vi "ping.vi"(7 "stop":bool, 8 "error in (no error)":errorcluster, 9 "Temperature (deg C)":dbl=25.0, 10 "myRIO DIO Channel":tag="C/DIO1", 11 "Digital in":refnum<vi>) -> (0 "error out":errorcluster, 3 "Distance (cm)":dbl)   [LabVIEW 2017]
uses:
  <vilib>/myRIO/Instrument Drivers/Onboard IO/DIO/typedefs/DIO Reference.ctl
  <vilib>/myRIO/Common/Instrument Driver Framework/Utilities/typedefs/myRIO Generic Hardware Reference.ctl
  <vilib>/myRIO/Common/Instrument Driver Framework/Utilities/typedefs/Hardware Version Enum.ctl
  <vilib>/myRIO/Common/Instrument Driver Framework/Utilities/typedefs/myRIO v1.0 Reference.ctl
  <vilib>/myRIO/Common/Instrument Driver Framework/Utilities/typedefs/Generic FPGA Reference.ctl
  <vilib>/myRIO/Common/Instrument Driver Framework/myRIO v1.0/DIO/typedefs/DIO Channels List.ctl
  <vilib>/myRIO/Common/Instrument Driver Framework/myRIO v1.0/DIO/typedefs/DIO Channels Enum.ctl
  <vilib>/userdefined/High Color/nirio_resource_hc.ctl
  <vilib>/myRIO/Common/Instrument Driver Framework/Utilities/vis/Is FPGA Ref Available.vi
  <vilib>/myRIO/Common/Instrument Driver Framework/myRIO v1.0/DIO/vis/myRIO v1.1 Open DIO.vi
  <vilib>/myRIO/Common/Instrument Driver Framework/Utilities/vis/Validate Channels.vi
  <vilib>/myRIO/Common/Instrument Driver Framework/myRIO v1.0/DIO/vis/myRIO v1.0 Reserve DIO.vi
  <vilib>/myRIO/Common/Instrument Driver Framework/myRIO v1.0/DIO/vis/myRIO v1.0 Close DIO.vi
  <vilib>/myRIO/Common/Instrument Driver Framework/myRIO v1.0/Resource Manager/vis/myRIO v1.0 Reserve Channel List.vi
  <vilib>/myRIO/Common/Instrument Driver Framework/myRIO v1.0/DIO/vis/myRIO v1.0 Build MUX Configuration DIO.vi
  <vilib>/myRIO/Common/Instrument Driver Framework/myRIO v1.0/DIO/vis/myRIO v1.0 Unreserve DIO.vi
  <vilib>/myRIO/Common/Instrument Driver Framework/myRIO v1.0/Resource Manager/vis/myRIO v1.0 Reserve Channel.vi
  <vilib>/myRIO/Common/Instrument Driver Framework/myRIO v1.0/Resource Manager/vis/myRIO v1.0 Unreserve Channel.vi
  <vilib>/myRIO/Common/Instrument Driver Framework/myRIO v1.0/Resource Manager/vis/myRIO v1.0 Create Configuration List.vi
  <vilib>/myRIO/Common/Instrument Driver Framework/myRIO v1.0/Resource Manager/vis/myRIO v1.0 Unreserve Channel List.vi
  <vilib>/myRIO/Common/Instrument Driver Framework/myRIO v1.0/Resource Manager/vis/myRIO v1.0 Build Mutex Name.vi
  <vilib>/Utility/VariantDataType/GetNumericInfo.vi
  <vilib>/Utility/error.llb/Error Cluster From Error Code.vi
  <vilib>/myRIO/Common/Instrument Driver Framework/myRIO v1.0/myRIO v1.1 Open.vi
  <vilib>/myRIO/Common/Instrument Driver Framework/Utilities/vis/IO Manager.vi
  <vilib>/myRIO/Common/Instrument Driver Framework/Utilities/vis/Configuration Manager.vi
  <vilib>/myRIO/Common/Instrument Driver Framework/myRIO v1.0/Resource Manager/vis/myRIO v1.0 Configure IO.vi
  <vilib>/myRIO/Common/Instrument Driver Framework/myRIO v1.0/myRIO v1.0 Close.vi
  <vilib>/myRIO/Common/Instrument Driver Framework/myRIO v1.0/DIO/vis/myRIO v1.0 Write DIO.vi
  <vilib>/myRIO/Common/Instrument Driver Framework/myRIO v1.0/DIO/vis/myRIO v1.0 Read DIO.vi
  <vilib>/myRIO/Common/Instrument Driver Framework/myRIO v1.0/DIO/vis/myRIO v1.0 Shutdown DIO.vi
  <vilib>/myRIO/Express VI/Onboard Devices/LED/LED Express VI.xnode
  <vilib>/myRIO/Instrument Drivers/Onboard IO/DIO/vis/myRIO DIO Open.xnode
  <vilib>/myRIO/Instrument Drivers/Onboard IO/DIO/DIO.lvlib
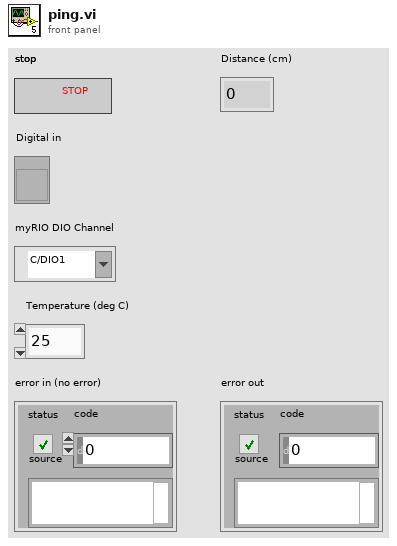
[diagram p1: front panel]
types:
  T1 = enum16{"Initialize", "Trigger pulse", "Wait for rising edge", "Wait for falling edge", "Calculate distance", "Stop"}
  T2 = typedef "DIO.lvlib/DIO Reference.ctl" = cluster{"myRIO Reference":T3, "DIO Channels List":T7}
  T3 = typedef "myRIO Generic Hardware Reference.ctl" = cluster{"myRIO Model":T4, "myRIO Hardware Reference":T5}
  T4 = typedef "Hardware Version Enum.ctl" = enum16{"Unknown", "myRIO-1900", "myRIO-1950", "roboRIO", "NI ELVIS RIO CM"}
  T5 = typedef "myRIO v1.0 Reference.ctl" = cluster{"Generic FPGA Reference":T6, "Allow multiple opens":bool}
  T6 = typedef "Generic FPGA Reference.ctl" = refnum<k20>
  T7 = typedef "DIO Channels List.ctl" = T8[]
  T8 = typedef "DIO Channels Enum.ctl" = enum16{"Not Connected", "C/DIO0", "C/DIO1", "C/DIO2", "C/DIO3", "C/DIO4", "C/DIO5", "C/DIO6", "C/DIO7", "A/DIO0", "A/DIO1", "A/DIO2", "A/DIO3", "A/DIO4", "A/DIO5", "A/DIO6", "A/DIO7", "A/DIO8", "A/DIO9", "A/DIO10", "A/DIO11", "A/DIO12", "A/DIO13", "A/DIO14", "A/DIO15", "B/DIO0", "B/DIO1", "B/DIO2", "B/DIO3", "B/DIO4", "B/DIO5", "B/DIO6", "B/DIO7", "B/DIO8", "B/DIO9", "B/DIO10", "B/DIO11", "B/DIO12", "B/DIO13", "B/DIO14", "B/DIO15", "LED0", "LED1", "LED2", "LED3", "Button0", "DIO/DIO0", "DIO/DIO1", "DIO/DIO2", "DIO/DIO3", "DIO/DIO4", "DIO/DIO5", "DIO/DIO6", "DIO/DIO7", "DIO/DIO8", "DIO/DIO9", "SPI/CS0", "SPI/CS1", "SPI/CS2", "SPI/CS3", "LED RADIO (Green)", "LED RADIO (Red)", "LED COMM (Green)", "LED COMM (Red)", "LED MODE (Green)", "LED MODE (Red)"}
  T9 = typedef "nirio_resource_hc.ctl" = tag
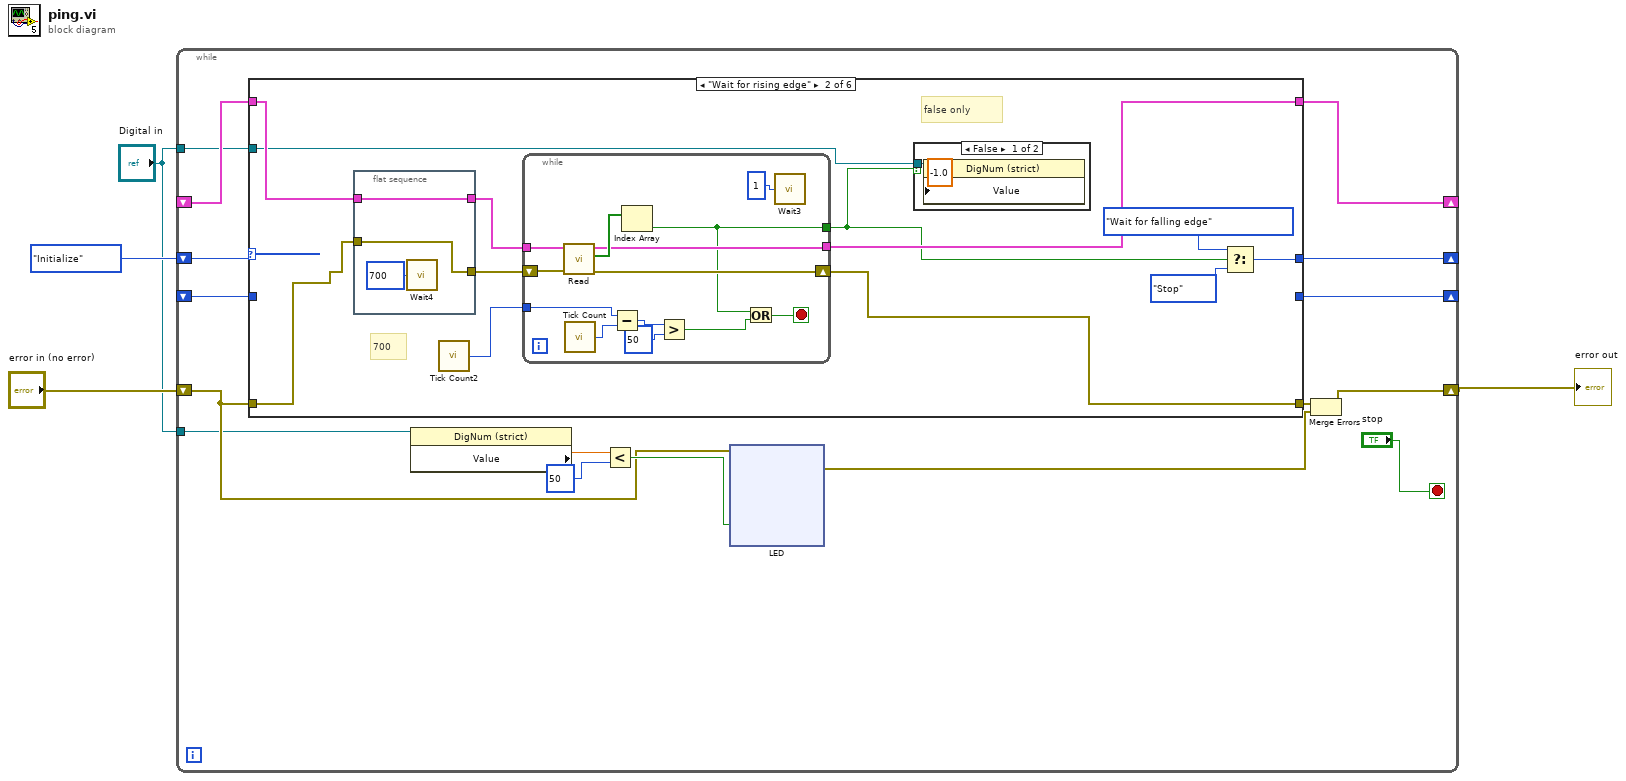
[diagram p0: block diagram]
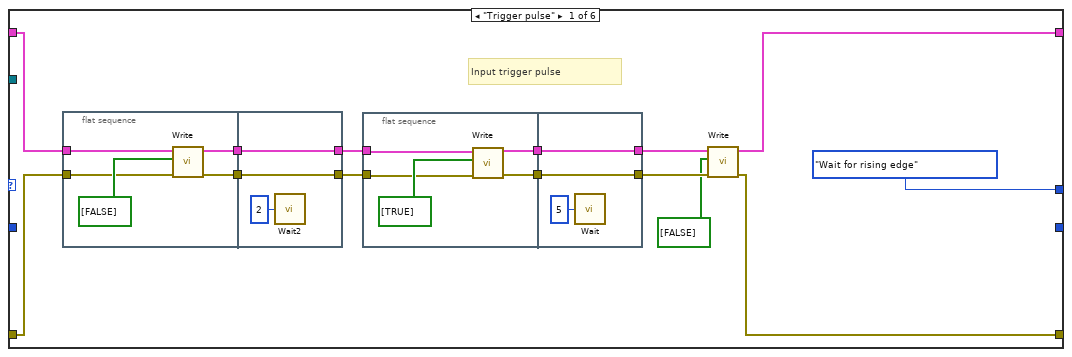
[diagram p2: hidden frame]
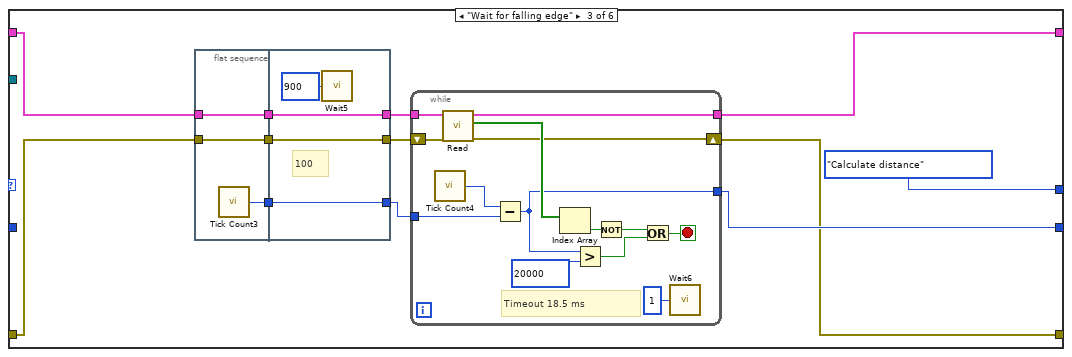
[diagram p4: hidden frame]
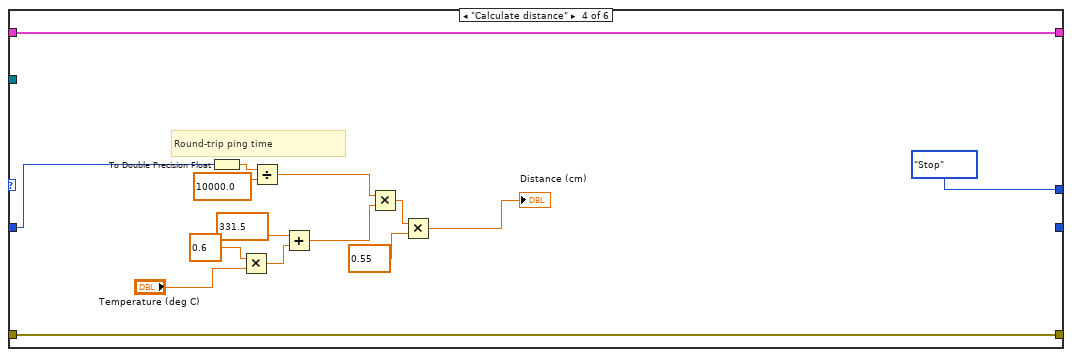
[diagram p5: hidden frame]
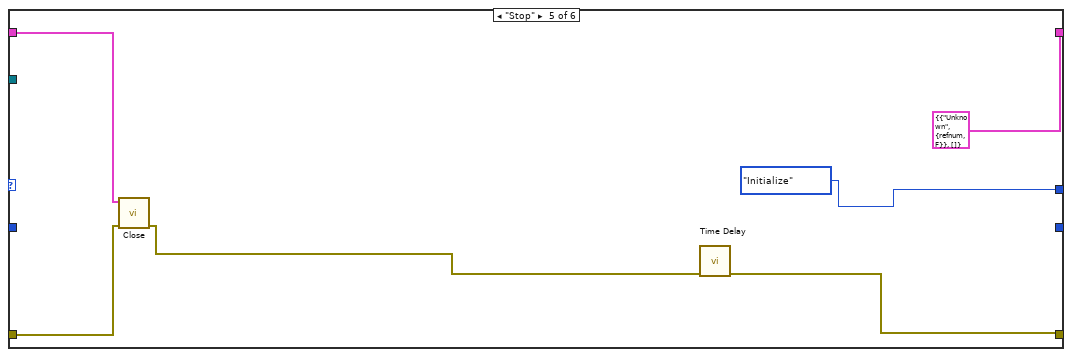
[diagram p6: hidden frame]
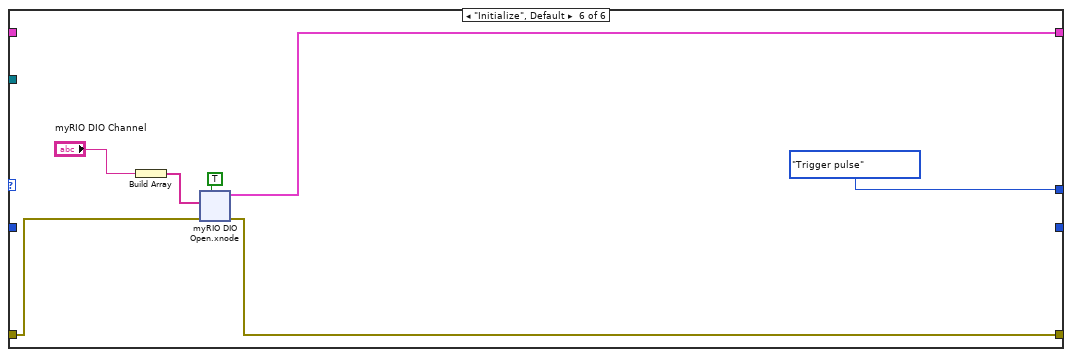
[diagram p7: hidden frame]
diagram:
  n1 = while {
    shift-right: [w15] -> _
    shift-left: T1."Initialize" -> [w20]
    shift-right: [w8] -> w4
    shift-left: "error in (no error)" -> [w9]
    shift-right: [w19] -> _
    shift-left: _ -> [w18]
    shift-right: [w14] -> _
    shift-left: _ -> [w16]
    tunnel: "Digital in" -> [w6]
    tunnel: "Digital in" -> [w5]
    stop <- "stop" stop-if-true
    n2 = case shown="\"Calculate distance\"" w20 {
      tunnel: [T1."Wait for rising edge" w53 T1."Calculate distance" ("y") T1."Stop" ("y") T1."Initialize" ("y") T1."Trigger pulse"] -> w15
      tunnel: w9 -> [w25 w58 w85 w116 w134 w139]
      tunnel: [w23 w62 w84 w128 T2 {"myRIO Reference"={"myRIO Model"=enum."Unknown", "myRIO Hardware Reference"={"Generic FPGA Reference"=refnum, "Allow multiple opens"=FALSE}}, "DIO Channels List"=[]} ("DIO Ref Out") w138] -> w19
      tunnel: w18 -> [w24 w57 w86 w128 w133 _]
      tunnel: [w22 w61 w81 w116 w129 w137] -> w17
      tunnel: [_ _ w83 _ _ _] -> w14
      tunnel: w16 -> [_ _ _ w115 _ _]
      tunnel: w6 -> [_ w51 _ _ _ _]
      frame "Trigger pulse" {
        # "Input trigger pulse"
        n3 = flat-sequence {
          tunnel: [w38] -> w32
          tunnel: [w37] -> w31
          tunnel: w25 -> [w36]
          tunnel: w24 -> [w35]
          tunnel: [w41] -> w29
          tunnel: [w40] -> w30
          tunnel: w32 -> [w41]
          tunnel: w31 -> [w40]
          frame #0 {
            n4 = call <vilib>:"Write.vi"("error in (no error)"=w36, "Values"=bool[] [FALSE], "DIO Ref In"=w35) -> ("error out"=w37:errorcluster, "DIO Ref Out"=w38:T2)  [unwired: 6 in]
          }
          frame #1 {
            n5 = call "Wait2"("Count(uSec)"=u32 2) -> ()  [unwired: 1 out]
          }
        }
        n6 = flat-sequence {
          tunnel: [w46] -> w34
          tunnel: [w45] -> w33
          tunnel: w30 -> [w44]
          tunnel: w29 -> [w43]
          tunnel: [w49] -> w26
          tunnel: [w48] -> w28
          tunnel: w34 -> [w49]
          tunnel: w33 -> [w48]
          frame #0 {
            n7 = call <vilib>:"Write.vi"("error in (no error)"=w44, "Values"=bool[] [TRUE], "DIO Ref In"=w43) -> ("error out"=w45:errorcluster, "DIO Ref Out"=w46:T2)  [unwired: 6 in]
          }
          frame #1 {
            n8 = call "Wait"("Count(uSec)"=u32 5) -> ()  [unwired: 1 out]
          }
        }
        n9 = call <vilib>:"Write.vi"("error in (no error)"=w28, "Values"=bool[] [FALSE], "DIO Ref In"=w26) -> ("error out"=w22:errorcluster, "DIO Ref Out"=w23:T2)  [unwired: 6 in]
      }
      frame "Wait for rising edge" {
        # "700"
        # "false only"
        n10 = flat-sequence {
          tunnel: [w66] -> w59
          tunnel: w58 -> [w66]
          tunnel: w57 -> [w65]
          tunnel: [w65] -> w56
          frame #0 {
            n11 = call "Wait4"("Count(uSec)"=u32 700) -> ()  [unwired: 1 out]
          }
        }
        n12 = call "Tick Count2"() -> ("Tick Count(uSec)"=w60:u32)
        n13 = while {
          tunnel: [w78] -> w62
          shift-right: [w76] -> w61
          shift-left: w59 -> [w77]
          tunnel: w60 -> [w73]
          tunnel: w56 -> [w75]
          tunnel: [w68] -> w52
          stop <- w70 stop-if-true
          n14 = call <vilib>:"Read.vi"("error in (no error)"=w77, "DIO Ref In"=w75) -> ("error out"=w76:errorcluster, "Values"=w79:bool[], "DIO Ref Out"=w78:T2)  [unwired: 7 in]
          n15 = call "Tick Count"() -> ("Tick Count(uSec)"=w74:u32)
          n16 = Subtract(x=w73, y=w74) -> (x-y=w72:u32)
          n17 = Index Array(array=w79) -> (element=w68:bool)  [unwired: 1 in]
          n18 = Greater?(x=w72, y=u32 50) -> (0:w69:bool)
          n19 = Or(x=w68, y=w69) -> (x .or. y?=w70:bool)
          n20 = call "Wait3"("Count(uSec)"=u32 1) -> ()  [unwired: 1 out]
        }
        n21 = case shown="False" w52 {
          tunnel: w51 -> [w63 _]
          frame False {
            n22 = property class="DigNum (strict)"(reference=w63, "Value"=-1.0 ("Distance (m)")) -> ()  [unwired: 1 in, 2 out]
          }
          frame True {
          }
        }
        n23 = Select(t=T1."Wait for falling edge", s=w52, f=T1."Stop" ("y")) -> (s? t:f=w53:T1)
      }
      frame "Wait for falling edge" {
        n24 = flat-sequence {
          tunnel: w86 -> [w109]
          tunnel: [w109] -> w92
          tunnel: [w108] -> w91
          tunnel: [w107] -> w90
          tunnel: w85 -> [w107]
          tunnel: [w112] -> w88
          tunnel: [w113] -> w89
          tunnel: w92 -> [w113]
          tunnel: w91 -> [w112]
          tunnel: w90 -> [w110]
          tunnel: [w110] -> w87
          frame #0 {
            n25 = call "Tick Count3"() -> ("Tick Count(uSec)"=w108:u32)
          }
          frame #1 {
            # "100"
            n26 = call "Wait5"("Count(uSec)"=u32 900) -> ()  [unwired: 1 out]
          }
        }
        n27 = while {
          tunnel: w89 -> [w105]
          tunnel: w88 -> [w102]
          shift-right: [w96] -> w81
          shift-left: w87 -> [w97]
          tunnel: [w94] -> w84
          tunnel: [w93] -> w83
          stop <- w101 stop-if-true
          # "Timeout 18.5 ms"
          n28 = call "Tick Count4"() -> ("Tick Count(uSec)"=w95:u32)
          n29 = call <vilib>:"Read.vi"("error in (no error)"=w97, "DIO Ref In"=w105) -> ("error out"=w96:errorcluster, "Values"=w104:bool[], "DIO Ref Out"=w94:T2)  [unwired: 7 in]
          n30 = Subtract(x=w95, y=w102) -> (x-y=w93:u32)
          n31 = Index Array(array=w104) -> (element=w103:bool)  [unwired: 1 in]
          n32 = Greater?(x=w93, y=u32 20000) -> (0:w99:bool)
          n33 = Not(x=w103) -> (.not. x?=w100:bool)
          n34 = Or(x=w100, y=w99) -> (x .or. y?=w101:bool)
          n35 = call "Wait6"("Count(uSec)"=u32 1) -> ()  [unwired: 1 out]
        }
      }
      frame "Calculate distance" {
        # "Round-trip ping time"
        n36 = To Double Precision Float(number=w115) -> (double precision float=w123:dbl)
        n37 = Multiply(x=0.6, y="Temperature (deg C)") -> (x*y=w121:dbl)
        n38 = Divide(x=w123, y=10000.0) -> (x/y=w125:dbl)
        n39 = Add(x=331.5, y=w121) -> (x+y=w126:dbl)
        n40 = Multiply(x=w125, y=w126) -> (x*y=w118:dbl)
        n41 = Multiply(x=w118, y=0.55) -> (x*y=→"Distance (cm)":dbl)
      }
      frame "Stop" {
        n42 = call <vilib>:"Close.vi"("error in (no error)"=w134, "DIO Ref In"=w133) -> ("error out"=w130:errorcluster)  [unwired: 9 in]
        n43 = call "Time Delay"("error in (no error)"=w130) -> ("error out"=w129:errorcluster)  [unwired: 10 in]
      }
      frame "Initialize", Default {
        n44 = Build Array("myRIO DIO Channel") -> (w141:tag[])
        n45 = xnode "myRIO DIO Open.xnode"("error in (no error)"=w139, "Allow multiple opens?"=TRUE, "Channel Names"=w141) -> ("error out"=w137:errorcluster, "DIO Ref Out"=w138:T2)
      }
    }
    n46 = property class="DigNum (strict)"(reference=w5) -> ("Value"=w12:dbl)  [unwired: 1 in, 2 out]
    n47 = Less?(x=w12, y=50) -> (x < y?=w10:bool)
    n48 = xnode "LED"("LED1"=w10, "error in (no error)"=w9) -> ("error out"=w7:errorcluster)
    n49 = Merge Errors(w17, w7) -> (w8:errorcluster)
  }
  "error out" <- w4
